vi "Choreo_EventMarker_FromJSON.vi"(11 "JSON String":string) -> (0 "Exists":bool, 3 "EventMarkers":T1[](array[typedef]))   [LabVIEW 2019, in "ChoreoLib.lvlib"]
doc: "Create a list of event markers from json string\n\nInputs:\n - JSONString - string - String potentially containing an event marker\n\nOutputs:\n - EventMarkers - array of cluster - The event markers defined by the given json object\n - Exists - boolean- TRUE if any event markers were found in the JSON string.\n\nNotes:\n--------\nCurrently the only type of commands that can be issued are Boolean commands. The value is forced to TRUE when the command is issued.\n\nThe following table lists the actions performed for different types of commands:\n - Unknown - nothing - not supported.\n - Wait - nothing - not supported\n - Named - Issue boolean command with TRUE value using the \"name\" as the command name.\n - Path - nothing - not supported\n - Sequential, Parallel, Race, Deadline - Issue boolean command with TRUE value for each of the commands contained in the \"commands\" array. The value for \"name\" is used as the command name."
uses:
  ChoreoLib.lvlib
  ENum/Choreo_Util_CommandType_ENUM.ctl
  TypeDef/ChoreoEventMarker.ctl
panel:
  in  "events":T2(array[cluster])
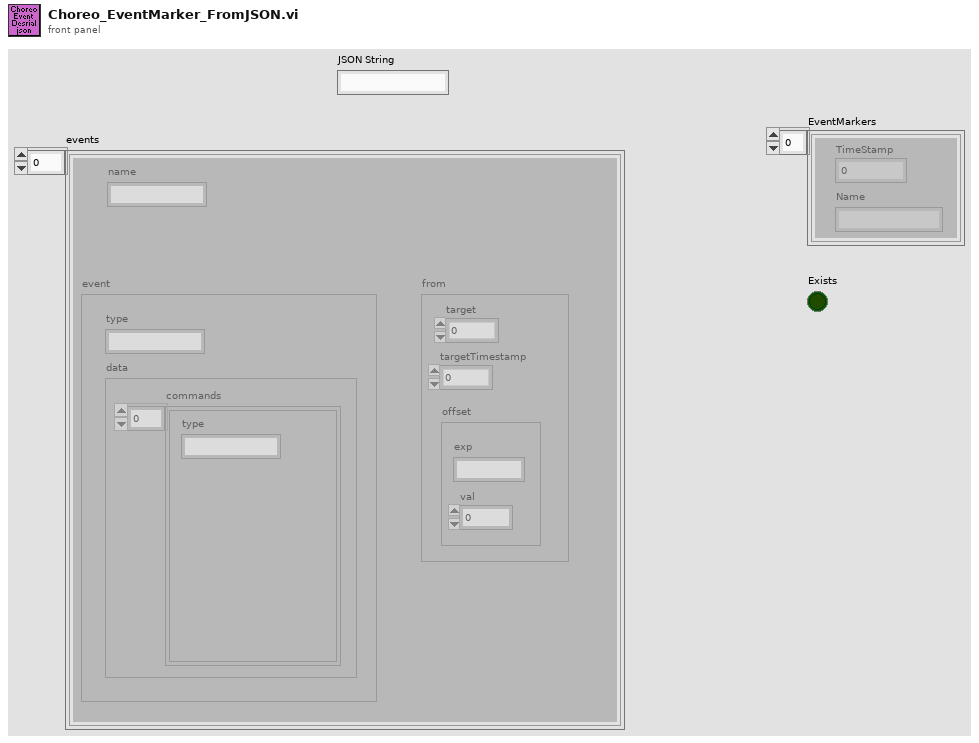
[diagram p1: front panel]
types:
  T1 = typedef "ChoreoLib.lvlib/ChoreoEventMarker.ctl" = cluster{"TimeStamp":dbl, "Name":string}
  T2 = cluster{"name":string, "event":cluster{"type":string, "data":cluster{"commands":cluster{"type":string}[]}}, "from":cluster{"targetTimestamp":dbl, "target":i32, "offset":cluster{"exp":string, "val":dbl}}}[]
  T3 = typedef "ChoreoLib.lvlib/Choreo_Util_CommandType_ENUM.ctl" = enum16{"Unknown", "Wait", "Named", "Path", "Sequential", "Parallel", "Race", "Deadline", "PointTowardsZoneEnter", "PointTowardsZoneExit", "TriggerEventStart", "TriggerEventStop", "TriggerEventOneshot"}
  T4 = cluster{"type":T3, "waitTime":dbl, "name":string, "pathName":string}
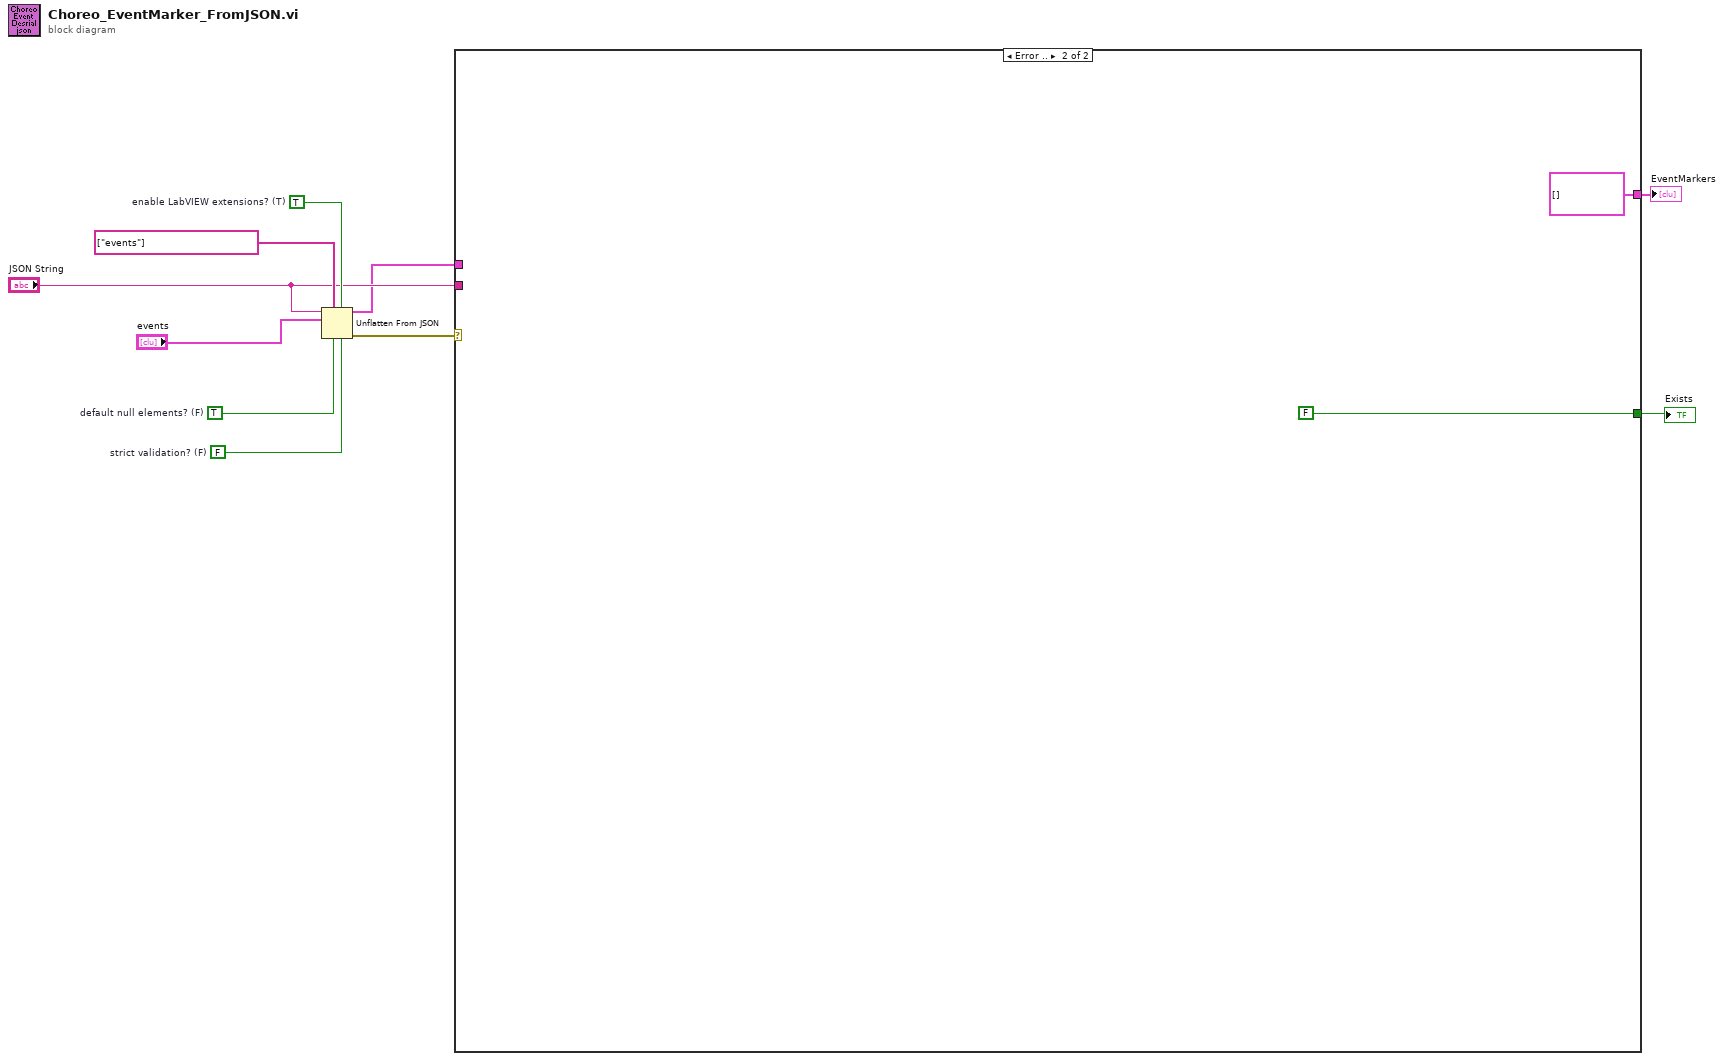
[diagram p0: block diagram]
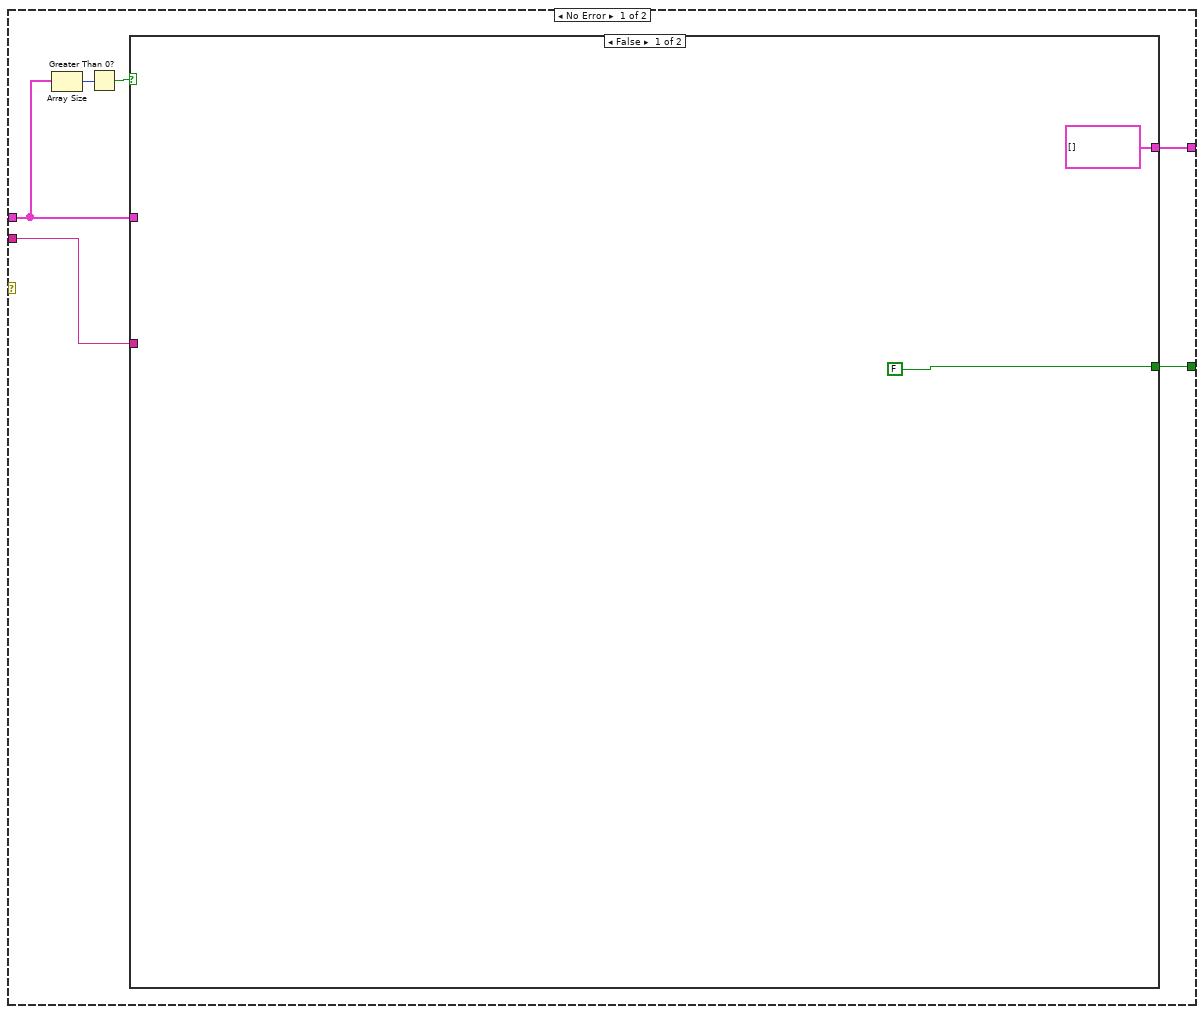
[diagram p2: hidden frame]
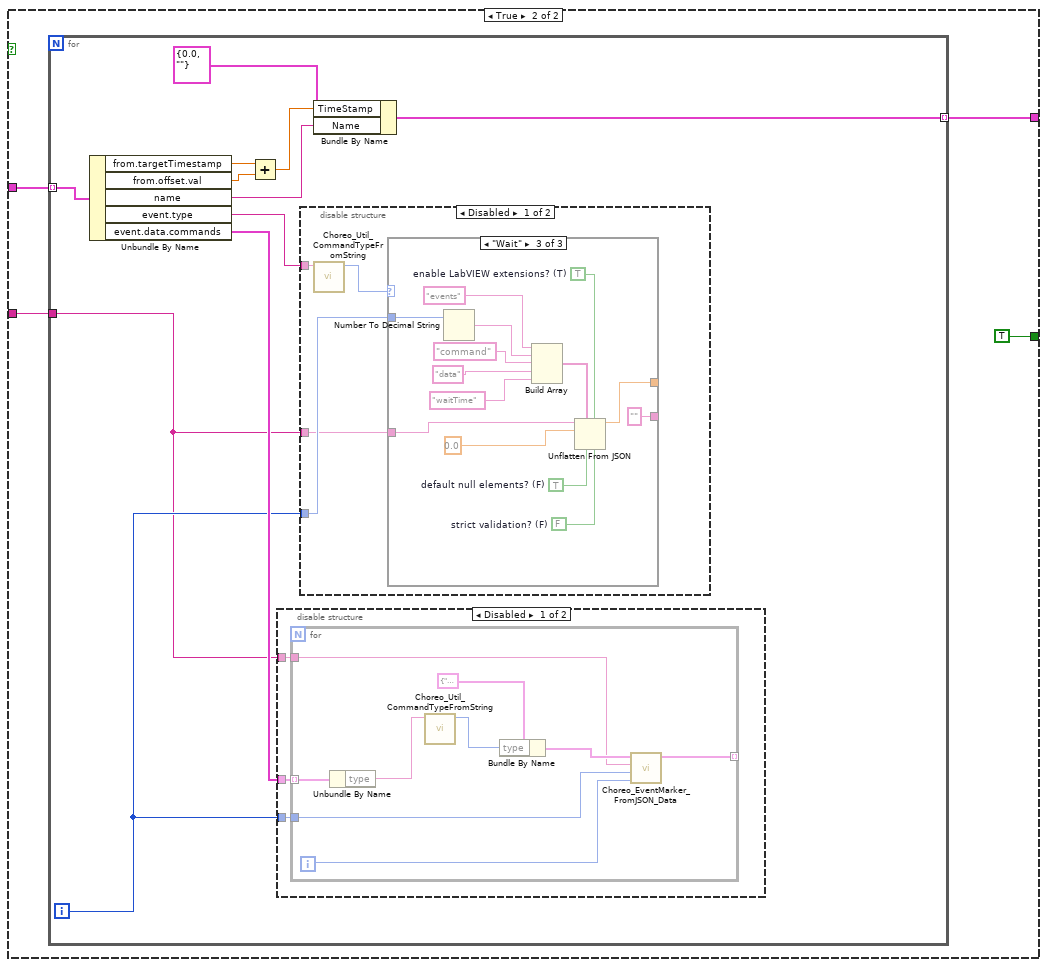
[diagram p3: hidden frame]
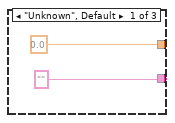
[diagram p5: hidden frame]
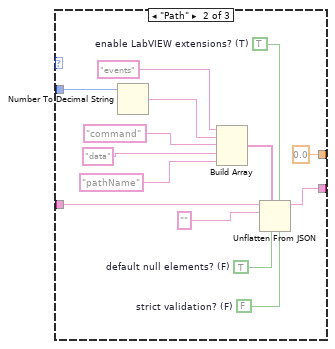
[diagram p6: hidden frame]
diagram:
  w7 = FALSE  # strict validation? (F)
  w8 = TRUE  # default null elements? (F)
  w9 = TRUE  # enable LabVIEW extensions? (T)
  n1 = Unflatten From JSON(path=string[] ["events"] ("path 2"), enable LabVIEW extensions? (T)=w9, JSON string="JSON String", type and defaults="events", default null elements? (F)=w8, strict validation? (F)=w7) -> (value=w2:T2, error out=w6:errorcluster)  [unwired: 1 in]
  n2 = case shown="Error .." w6 {
    tunnel: [w14 FALSE] -> w4
    tunnel: "JSON String" -> [w13 _]
    tunnel: w2 -> [w12 _]
    tunnel: [w11 T1[] []] -> w1
    frame No Error {
      n3 = Array Size(array=w12) -> (size(s)=w16:i32)
      n4 = Greater Than 0?(x=w16) -> (x > 0?=w15:bool)
      n5 = case shown="False" w15 {
        tunnel: [FALSE TRUE] -> w14
        tunnel: w13 -> [_ w21]
        tunnel: w12 -> [_ w20]
        tunnel: [T1[] [] w19] -> w11
        frame False {
        }
        frame True {
          n6 = for {
            tunnel: w20 -> [w33] mode=indexing
            tunnel: w21 -> [w29]
            tunnel: [w23] -> w19 mode=indexing
            i -> [w30]
            n7 = Unbundle By Name(w33) -> ("from.targetTimestamp"=w26:dbl, "from.offset.val"=w27:dbl, "name"=w24:string, "event.type"=w31:string, "event.data.commands"=w32:cluster{"type":string}[])
            n8 = Add(x=w26, y=w27) -> (x+y=w25:dbl)
            n9 = disable-structure shown="Disabled" {
              disable-tunnel: w32 -> [w36 _]
              disable-tunnel: w30 -> [w35 _]
              disable-tunnel: w29 -> [w34 _]
              frame Disabled {
                n10 = for {
                  tunnel: w36 -> [w45] mode=indexing
                  tunnel: [w40] -> _ mode=indexing
                  tunnel: w34 -> [w39]
                  tunnel: w35 -> [w38]
                  i -> [w37]
                  n11 = Unbundle By Name(w45) -> ("type"=w43:string)
                  n12 = call "Choreo_Util_CommandTypeFromString.vi"("Type string"=w43) -> ("Type"=w44:T3)  [unwired: 10 in]
                  n13 = Bundle By Name(cluster=T4 {"type"=enum."Unknown", "waitTime"=0.0, "name"="", "pathName"=""} ("Command"), "type"=w44) -> (w41:T4)
                  n14 = call "Choreo_EventMarker_FromJSON_Data.vi"("Cmd Index"=w37, "Index"=w38, "JSON String"=w39, "In Command Data"=w41) -> ("out Command Data"=w40:T4)  [unwired: 6 in, 1 out]
                }
              }
              frame Enabled {
              }
            }
            n15 = disable-structure shown="Disabled" {
              disable-tunnel: w31 -> [w49 _]
              disable-tunnel: w30 -> [w47 _]
              disable-tunnel: w29 -> [w46 _]
              frame Disabled {
                n16 = call "Choreo_Util_CommandTypeFromString.vi"("Type string"=w49) -> ("Type"=w48:T3)  [unwired: 10 in]
                n17 = case shown="\"Wait\"" w48 {
                  tunnel: w46 -> [_ w61 w72]
                  tunnel: ["" w56 ""] -> _
                  tunnel: [0.0 0.0 w70] -> _
                  tunnel: w47 -> [_ w53 w68]
                  frame "Unknown", Default {
                  }
                  frame "Path" {
                    w63 = FALSE  # strict validation? (F)
                    w64 = TRUE  # default null elements? (F)
                    w65 = TRUE  # enable LabVIEW extensions? (T)
                    n18 = Number To Decimal String(number=w53) -> (decimal integer string=w52:string)  [unwired: 1 in]
                    n19 = Build Array("events", w52, "command", "data", "pathName") -> (w60:string[])
                    n20 = Unflatten From JSON(path=w60, enable LabVIEW extensions? (T)=w65, JSON string=w61, type and defaults="", default null elements? (F)=w64, strict validation? (F)=w63) -> (value=w56:string)  [unwired: 1 in, 1 out]
                  }
                  frame "Wait" {
                    w77 = FALSE  # strict validation? (F)
                    w78 = TRUE  # default null elements? (F)
                    w79 = TRUE  # enable LabVIEW extensions? (T)
                    n21 = Number To Decimal String(number=w68) -> (decimal integer string=w67:string)  [unwired: 1 in]
                    n22 = Build Array("events", w67, "command", "data", "waitTime") -> (w76:string[])
                    n23 = Unflatten From JSON(path=w76, enable LabVIEW extensions? (T)=w79, JSON string=w72, type and defaults=0.0, default null elements? (F)=w78, strict validation? (F)=w77) -> (value=w70:dbl)  [unwired: 1 in, 1 out]
                  }
                }
              }
              frame Enabled {
              }
            }
            n24 = Bundle By Name(cluster=T1 {"TimeStamp"=0.0, "Name"=""} ("ChoreoEvent"), "TimeStamp"=w25, "Name"=w24) -> (w23:T1)
          }
        }
      }
    }
    frame Error {
    }
  }
  "Exists" <- w4
  "EventMarkers" <- w1
